vi "Steady-State Error.vi"() -> ()   [LabVIEW 2018]
uses:
  <vilib>/Simulation/Scripting/Companion Diagram/SimConfigNode/SimParams.ctl
  <vilib>/Simulation/Scripting/Companion Diagram/SimConfigNode/_simSolvers.ctl
  <vilib>/Simulation/Implementation/Shared/SIMSCR Execution Mode.ctl
  <vilib>/Platform/TimedLoop/XDataNode/timing_clust.ctl
  <vilib>/Platform/TimedLoop/XDataNode/nitl_modes.ctl
  <vilib>/Platform/TimedLoop/XDataNode/wakeup.ctl
  <vilib>/Simulation/Param Hierarchy/Typedefs/SIMPH Param Control Actions.ctl
  <vilib>/Simulation/Implementation/Shared/NILVSim_ParamChanged.vi
  <vilib>/Simulation/Implementation/Shared/NILVSim_FinishedLate.vi
  <vilib>/Simulation/Implementation/Shared/NILVSIM_BeginStep.vi
  <vilib>/Simulation/Utility/Implementation/SIM Halt.vi
  <vilib>/Simulation/ContinuousLinear/Implementation/NILVSim Transfer Function Direct.llb/SIM Transfer Function Direct (SISO).vi
  <vilib>/Simulation/Utility/Implementation/SIM Time.vi
  <vilib>/Simulation/SignalDisplay/Implementation/NILVSim Time Waveform.llb/SIM Time Waveform (vector).vi
  <vilib>/Simulation/Nonlinear/Implementation/NILVSim Saturation.llb/SIM Saturation (scalar).vi
  <vilib>/Simulation/SignalDisplay/Implementation/NILVSim Time Waveform.llb/SIM Time Waveform (scalar).vi
  <vilib>/Simulation/Implementation/Shared/NILVSim_Manager.vi
  <vilib>/Utility/error.llb/Clear Errors.vi
  <vilib>/Simulation/Implementation/Shared/NILVSim_FinalizeModel.vi
  <vilib>/Simulation/Implementation/Shared/SIM Unbundle Sim Info.vi
  <vilib>/Simulation/Implementation/Shared/SIMSH Read Queue.vi
  <vilib>/Simulation/Implementation/Shared/NILVSim_Initialize.vi
  SubVIs/Encoders.vi
  <vilib>/Simulation/Utility/Implementation/NILVSim Get Time and IsAcceptedStep.vi
  <vilib>/ptbypt/Signal Generation.llb/Triangle Wave PtByPt.vi
  SubVIs/Motor.vi
  <vilib>/Simulation/Implementation/Shared/NILVSim_GetModelError.vi
  <vilib>/Simulation/Implementation/Shared/SIM Bundle Sim Info.vi
  <vilib>/Simulation/Scripting/Companion Diagram/SimConfigNode/SimDog.xnode
  SubVIs/PID_Control.vi
  <vilib>/Platform/TimedLoop/XDataNode/XDataNode.xnode
  <vilib>/Simulation/Implementation/XNodeFramework/SimXNode/SimX.xnode
  <vilib>/ptbypt/NI_PtbyPt.lvlib
  <vilib>/Platform/TimedLoop/XDataNode/XDNodeRunTimeDep.lvlib
  <vilib>/Simulation/Implementation/Shared/NI_SIM_Implementation.lvlib
panel:
  in  "Stop Button":bool
  in  "Control Parameters":cluster{"kp":dbl, "kd":dbl, "ki":dbl}={"kp"=1.0, "kd"=0.0, "ki"=0.0} {"ki" step=0.05; "kd" step=0.05; "kp" step=0.005}
  in  "Signal Generator (ramp)":T1={"Amplitude (rad)"=5.0, "Frequency (Hz)"=0.2} {"Frequency (Hz)" step=0.1}
  out "Motor Voltage":waveform(dbl)(graph)={"t0"=timestamp(19.19 s since 1904-01-01), "dt"=1.0, "Y"=[1.7574388110467847]}
  out "Motor Position":waveform(dbl)[](graph)=[{"t0"=timestamp(19.19 s since 1904-01-01), "dt"=1.0, "Y"=[40.0]}, {"t0"=timestamp(19.19 s since 1904-01-01), "dt"=1.0, "Y"=[40.39795078767929]}]
  out "Error":errorcluster={"status"=FALSE, "code"=-363017, "source"="ELVIS III v1.0 Write PWM.vi"}
  # "Engineering Trainer Boards"
  # "Controls Board"
  # "Steady-State Error"
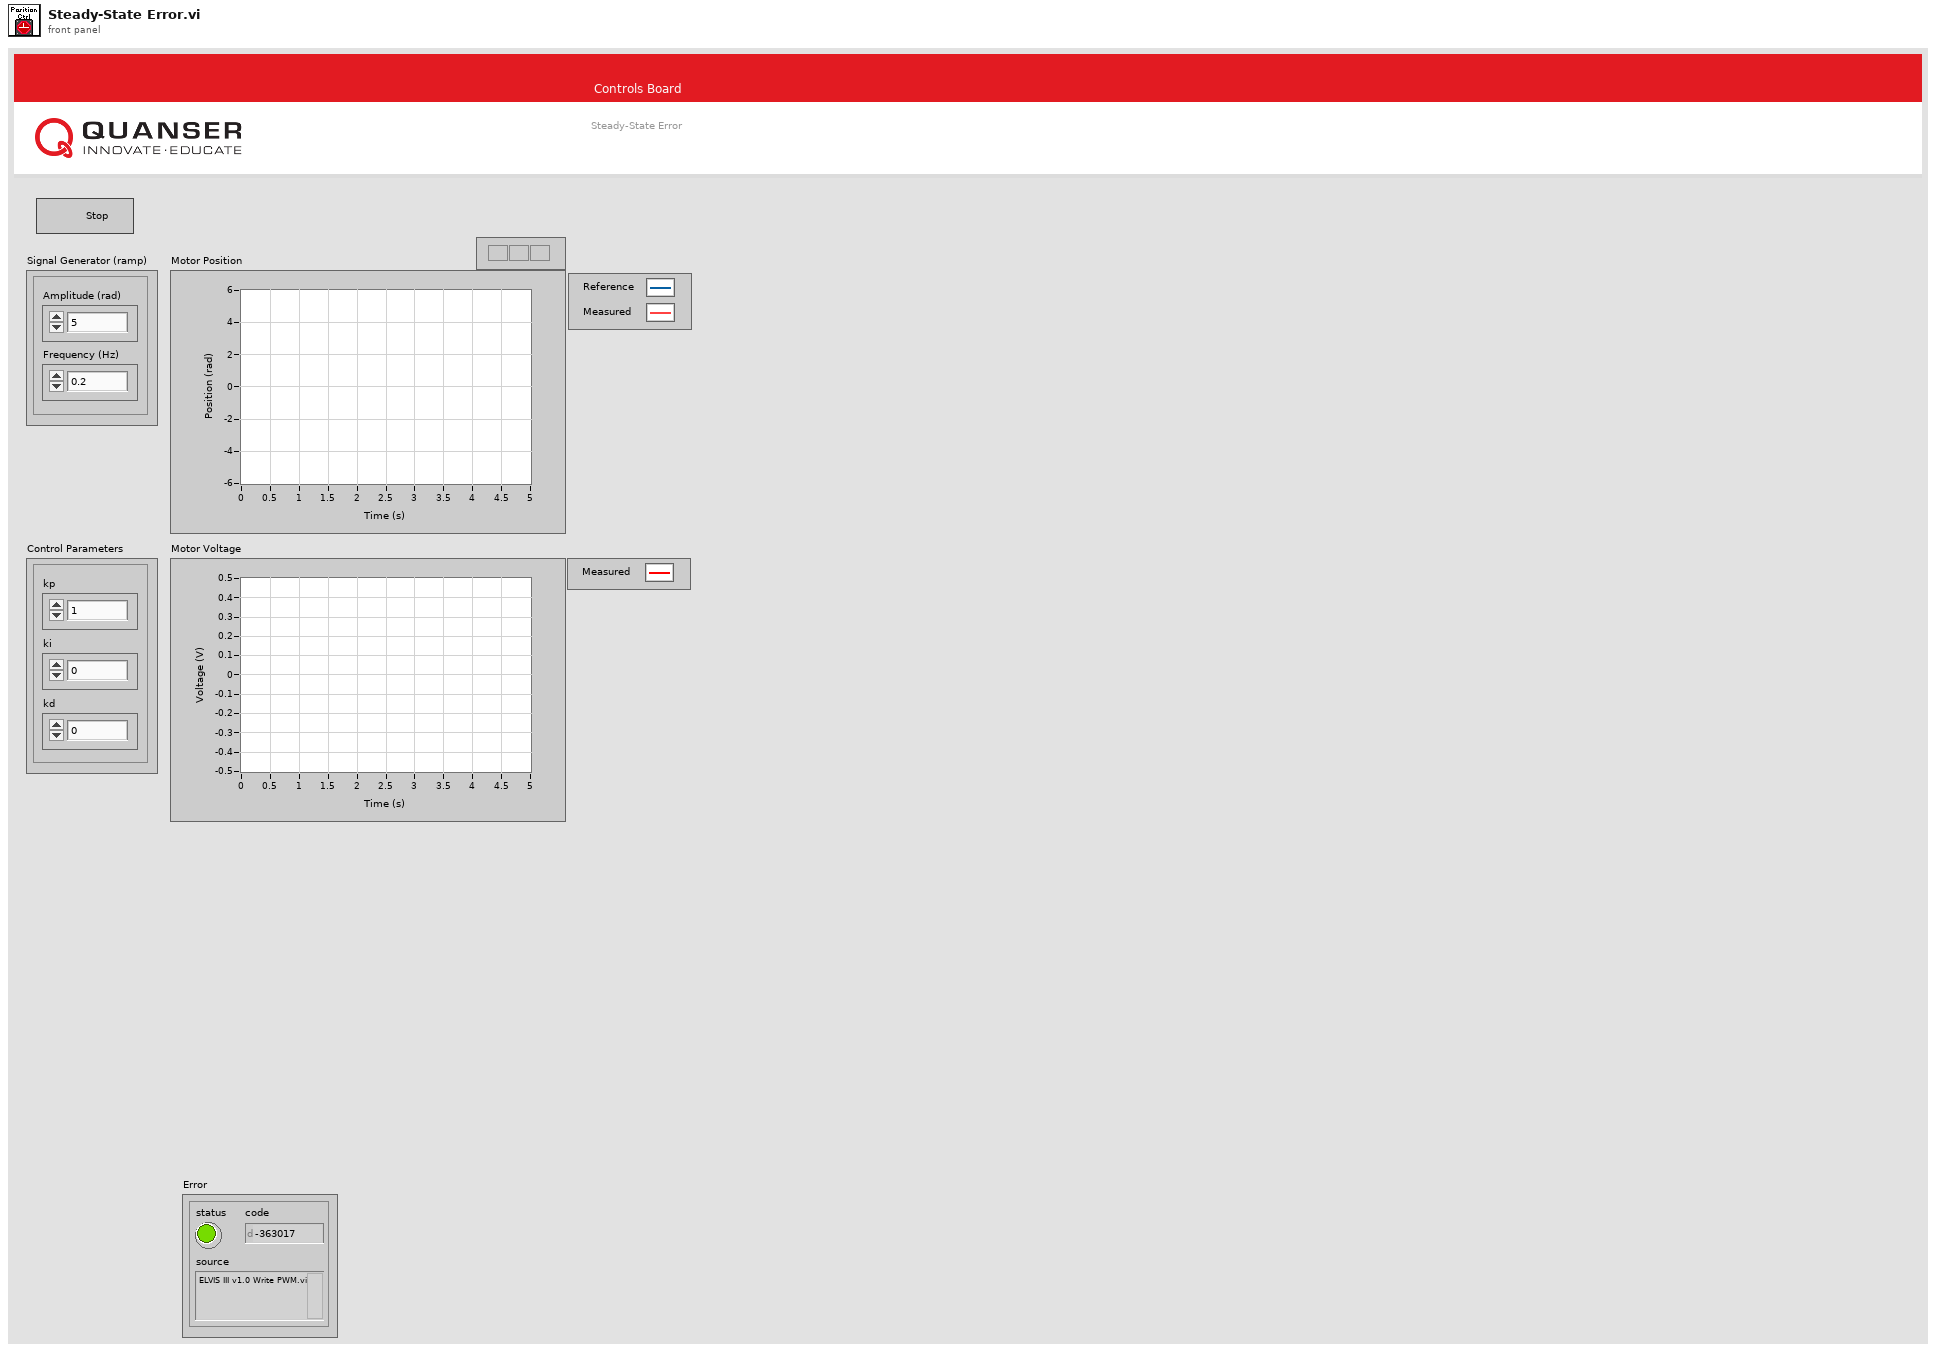
[diagram p1: front panel]
types:
  T1 = cluster{"Amplitude (rad)":dbl, "Frequency (Hz)":dbl}
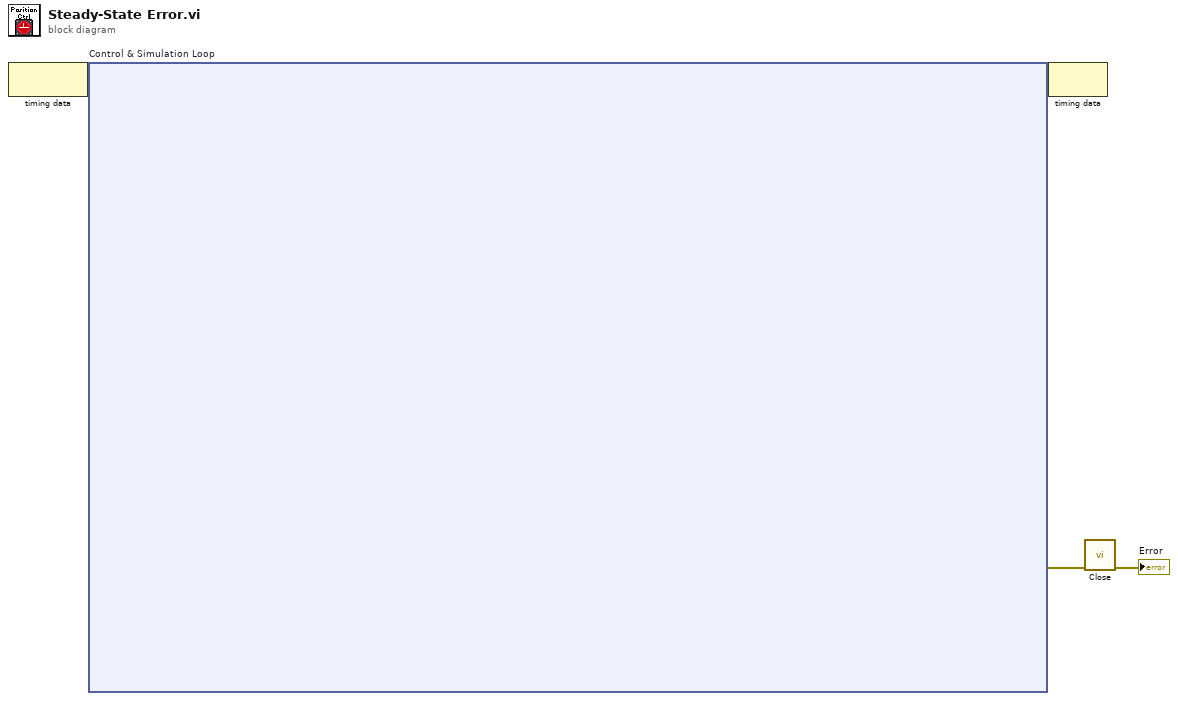
[diagram p0: block diagram]
diagram:
  n1 = node-c288() -> (w4:variant)  [unwired: 1 in]
  n2 = node-c254 "Control & Simulation Loop"(w4) -> (w3:variant, w2:errorcluster)
  n3 = node-c288(w3) -> ()  [unwired: 1 out]
  n4 = call "Close.vi"("error in"=w2) -> ("error out"=→"Error":errorcluster)  [unwired: 10 in]
